vi "Compile Analog Replay 1.0 Data.vi"(8 "error in (no error)":errorcluster, 11 "Device Item Ref in":T3 format="%.0x") -> (0 "error out":errorcluster, 1 "bitfile names":string[](array[string]), 2 "Analog Replays":T1[](array[typedef]), 3 "Device Item Ref out":T3 format="%.0x")   [LabVIEW 2015, in "Engine Simulation Toolkit System Explorer.lvlib"]
uses:
  Engine Simulation Toolkit System Explorer.lvlib
  <vilib>/NI Veristand/Custom Device API/Custom Device Item Ref.ctl
  Shared/1.0 Analog Replay Engine Data.ctl
  Shared/1.0 Analog Replay FIFO Idxs.ctl
  Position Reference.ctl
  Shared/Properties.vi
  Shared/Constants and GUIDs.vi
  <vilib>/NI Veristand/Custom Device Tools/Custom Device Utility Library/NI VeriStand - Search for All Items by GUID.vi
  <vilib>/NI Veristand/Custom Device API/Get Item Property (String).vi
  <vilib>/NI Veristand/Custom Device API/Get Item Property (Boolean).vi
  <vilib>/NI Veristand/Custom Device API/Get Item Property (U16).vi
  <vilib>/NI Veristand/Custom Device API/Get Item Property (Double).vi
  Shared/Engine Simulation Toolkit Shared.lvlib
  <vilib>/NI Veristand/Custom Device API/Custom Device API.lvlib
  <vilib>/NI Veristand/Custom Device Tools/Custom Device Utility Library/Custom Device Utility Library.lvlib
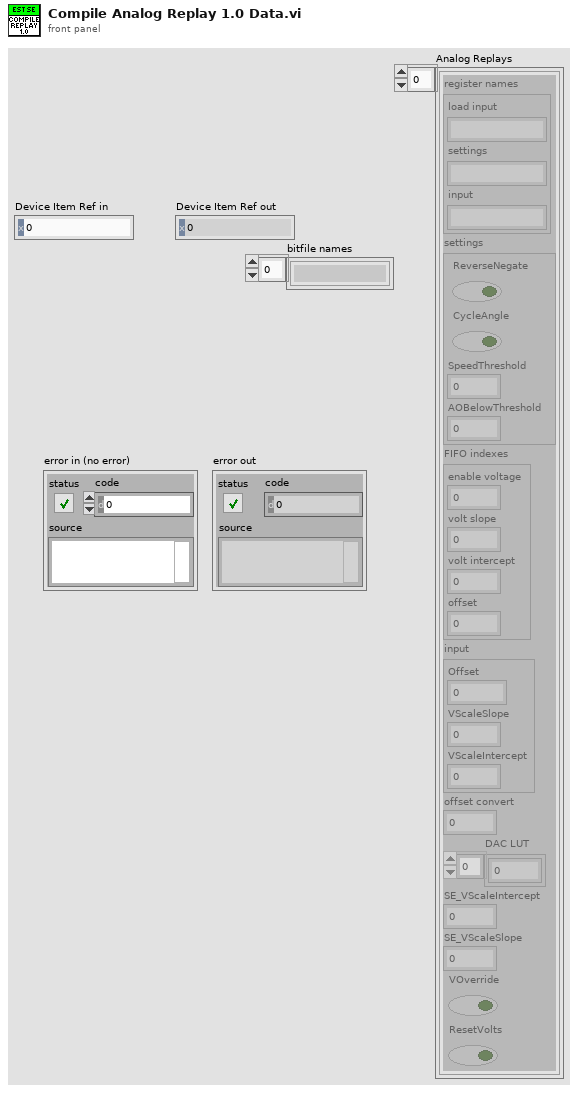
[diagram p1: front panel]
types:
  T1 = typedef "Engine Simulation Toolkit Shared.lvlib/1.0 Analog Replay Engine Data.ctl" = cluster{"register names":cluster{"load input":string, "settings":string, "input":string}, "settings":cluster{"ReverseNegate":bool, "CycleAngle":bool, "SpeedThreshold":fxp<+/-,23,2>, "AOBelowThreshold":i16}, "FIFO indexes":T2, "input":cluster{"Offset":i16, "VScaleSlope":fxp<+,18,6>, "VScaleIntercept":fxp<+/-,18,3>}, "offset convert":dbl, "DAC LUT":i16[], "SE_VScaleIntercept":fxp<+/-,18,3>, "SE_VScaleSlope":fxp<+,18,6>, "VOverride":bool, "ResetVolts":bool}
  T2 = typedef "Engine Simulation Toolkit Shared.lvlib/1.0 Analog Replay FIFO Idxs.ctl" = cluster{"enable voltage":i32, "volt slope":i32, "volt intercept":i32, "offset":i32}
  T3 = typedef "Custom Device API.lvlib/Custom Device Item Ref.ctl" = u64
  T4 = typedef "Engine Simulation Toolkit System Explorer.lvlib/Position Reference.ctl" = enum16{"Crank angle", "Cycle angle"}
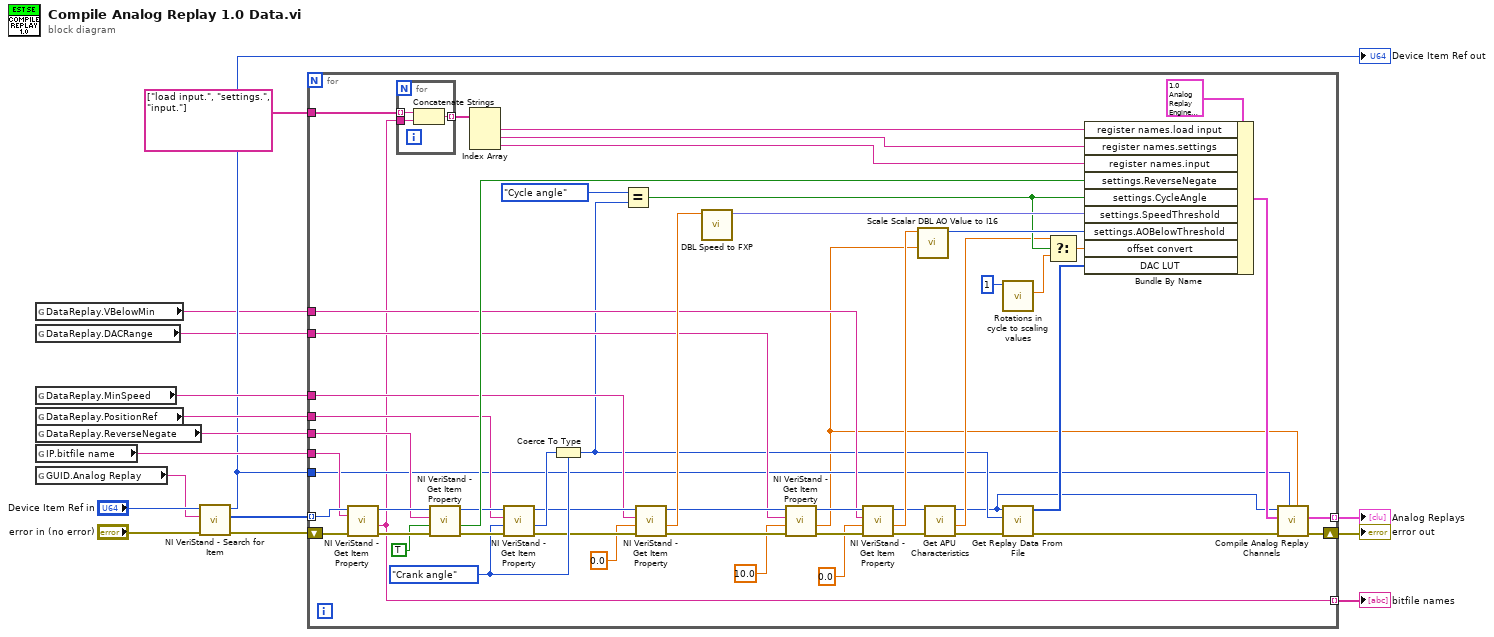
[diagram p0: block diagram]
diagram:
  n1 = global read "Properties.vi" "DataReplay.VBelowMin"() -> (w3:string)
  n2 = global read "Properties.vi" "DataReplay.DACRange"() -> (w4:string)
  n3 = global read "Properties.vi" "DataReplay.MinSpeed"() -> (w7:string)
  n4 = global read "Properties.vi" "DataReplay.PositionRef"() -> (w8:string)
  n5 = global read "Properties.vi" "DataReplay.ReverseNegate"() -> (w10:string)
  n6 = global read "Properties.vi" "IP.bitfile name"() -> (w12:string)
  n7 = global read "Constants and GUIDs.vi" "GUID.Analog Replay"() -> (w14:string)
  n8 = call-poly <vilib>:"NI VeriStand - Search for Item.vi"("error in"="error in (no error)", "Item GUID"=w14, "Section Ref in"="Device Item Ref in") -> ("error out"=w13:errorcluster, "Item Refs"=w5:T3[], "Section Ref out"=w6:T3)  [unwired: 5 in, 1 out]
  "Device Item Ref out" <- w6
  n9 = for {
    shift-right: [w25] -> w9
    shift-left: w13 -> [w70]
    tunnel: w5 -> [w69] mode=indexing
    tunnel: w12 -> [w68]
    tunnel: string[] ["load input.", "settings.", "input."] -> [w67]
    tunnel: w10 -> [w60]
    tunnel: w8 -> [w55]
    tunnel: w7 -> [w48]
    tunnel: w6 -> [w20]
    tunnel: w4 -> [w42]
    tunnel: w3 -> [w38]
    tunnel: [w22] -> w2 mode=indexing
    tunnel: [w17] -> w1 mode=indexing
    w54 = Position_Reference."Crank angle" ("Position reference")
    n10 = call-poly <vilib>:"NI VeriStand - Get Item Property.vi"("error in (no error)"=w70, "Property Name"=w68, "Item Ref in"=w69) -> ("error out"=w61:errorcluster, "Value"=w17:string, "Item Ref out"=w62:T3)  [unwired: 5 in, 1 out]
    n11 = for {
      tunnel: w17 -> [w73]
      tunnel: w67 -> [w72] mode=indexing
      tunnel: [w71] -> w65 mode=indexing
      n12 = Concatenate Strings(w72, w73) -> (w71:string)
    }
    n13 = call-poly <vilib>:"NI VeriStand - Get Item Property.vi"("error in (no error)"=w61, "Default Value"=TRUE, "Property Name"=w60, "Item Ref in"=w62) -> ("error out"=w56:errorcluster, "Value"=w59:bool, "Item Ref out"=w57:T3)  [unwired: 4 in, 1 out]
    n14 = Index Array(array=w65) -> (element #1=w64:string, element #2=w63:string, element #3=w19:string)  [unwired: 3 in]
    n15 = call-poly <vilib>:"NI VeriStand - Get Item Property.vi"("error in (no error)"=w56, "Default Value"=w54, "Property Name"=w55, "Item Ref in"=w57) -> ("error out"=w51:errorcluster, "Value"=w53:u16, "Item Ref out"=w49:T3)  [unwired: 4 in, 1 out]
    n16 = Coerce To Type(0:w53, 1:w54) -> (2:w28:T4)
    n17 = Equal?(x=Position_Reference."Cycle angle" ("Position reference"), y=w28) -> (x = y?=w33:bool)
    n18 = call-poly <vilib>:"NI VeriStand - Get Item Property.vi"("error in (no error)"=w51, "Default Value"=0.0, "Property Name"=w48, "Item Ref in"=w49) -> ("error out"=w50:errorcluster, "Value"=w47:dbl, "Item Ref out"=w44:T3)  [unwired: 4 in, 1 out]
    n19 = call "DBL Speed to FXP.vi"("Desired speed (RPM)"=w47) -> ("FXP speed"=w45:fxp<+/-,23,2>)  [unwired: 6 in, 4 out]
    n20 = call-poly <vilib>:"NI VeriStand - Get Item Property.vi"("error in (no error)"=w50, "Default Value"=10.0, "Property Name"=w42, "Item Ref in"=w44) -> ("error out"=w43:errorcluster, "Value"=w18:dbl, "Item Ref out"=w39:T3)  [unwired: 4 in, 1 out]
    n21 = call-poly <vilib>:"NI VeriStand - Get Item Property.vi"("error in (no error)"=w43, "Default Value"=0.0, "Property Name"=w38, "Item Ref in"=w39) -> ("error out"=w40:errorcluster, "Value"=w36:dbl, "Item Ref out"=w34:T3)  [unwired: 4 in, 1 out]
    n22 = call "Scale Scalar DBL AO Value to I16.vi"("DAC bipolar range"=w18, "AO DBL value"=w36) -> ("AO I16 value"=w35:i16)  [unwired: 9 in]
    n23 = call "Get APU Characteristics.vi"("error in (no error)"=w40, "Item Ref in"=w34) -> ("error out"=w27:errorcluster, "angle to u16 scale factor"=w31:dbl, "Item Ref out"=w21:T3)  [unwired: 3 in, 4 out]
    n24 = call "Rotations in cycle to scaling values.vi"("rotations in a cycle"=u16 1) -> ("angle to u16 scale factor"=w30:dbl)  [unwired: 8 in, 2 out]
    n25 = call "Get Replay Data From File.vi"("error in (no error)"=w27, "Position reference"=w28, "Item Ref in"=w21) -> ("error out"=w24:errorcluster, "DAC Data"=w26:i16[])  [unwired: 6 in, 1 out]
    n26 = Select(t=w31, s=w33, f=w30) -> (s? t:f=w29:dbl)
    n27 = Bundle By Name(cluster=T1 {"register names"={"load input"="", "settings"="", "input"=""}, "settings"={"ReverseNegate"=FALSE, "CycleAngle"=FALSE, "SpeedThreshold"=0.0, "AOBelowThreshold"=0}, "FIFO indexes"={"enable voltage"=0, "volt slope"=0, "volt intercept"=0, "offset"=0}, "input"={"Offset"=0, "VScaleSlope"=0.0, "VScaleIntercept"=0.0}, "offset convert"=0.0, "DAC LUT"=[], "SE_VScaleIntercept"=0.0, "SE_VScaleSlope"=0.0, "VOverride"=FALSE, "ResetVolts"=FALSE} ("1.0.0 Analog Replay"), "register names.load input"=w64, "register names.settings"=w63, "register names.input"=w19, "settings.ReverseNegate"=w59, "settings.CycleAngle"=w33, "settings.SpeedThreshold"=w45, "settings.AOBelowThreshold"=w35, "offset convert"=w29, "DAC LUT"=w26) -> (w23:T1)
    n28 = call "Compile Analog Replay Channels.vi"("DAC bipolar range"=w18, "Custom device ref"=w20, "error in (no error)"=w24, "1.0.0 Analog Replay in"=w23, "Item Ref in"=w21) -> ("error out"=w25:errorcluster, "1.0.0 Analog Replay out"=w22:T1)  [unwired: 5 in]
  }
  "error out" <- w9
  "Analog Replays" <- w2
  "bitfile names" <- w1
